vi "Mag Lab Init Device List.vi"(8 "error in (no error)":errorcluster) -> (0 "error out":errorcluster, 2 "find list":refnum<visa-resource-name>[](array[refnum]), 3 "Found Array":refnum<class "Mag Lab Hardware.lvclass">[](array[class]))   [LabVIEW 2015]
uses:
  Mag Lab Hardware.lvclass
  <vilib>/Instr/_visa.llb/VISA Find Search Mode.ctl
panel:
  out "Names":string[](array[string])
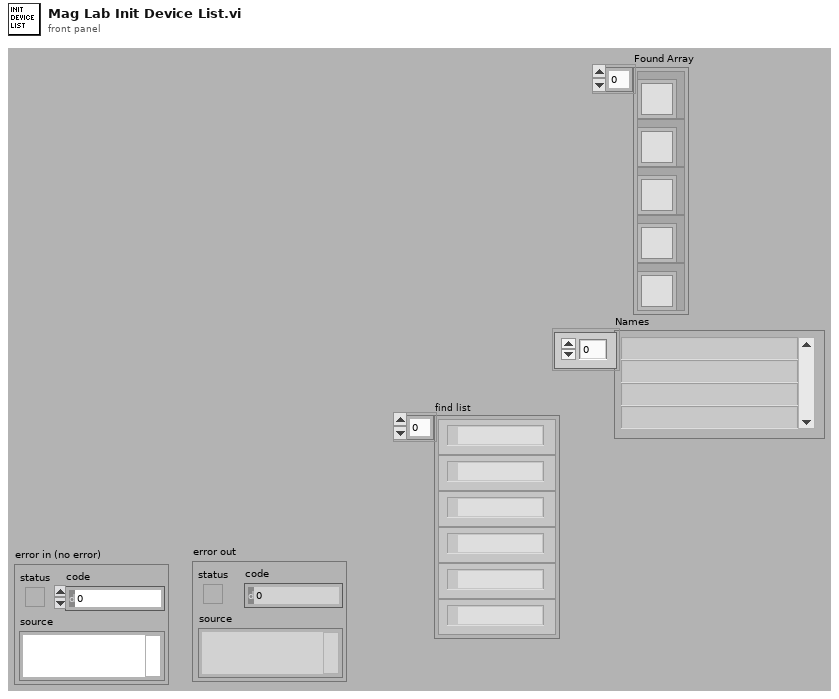
[diagram p1: front panel]
types:
  T1 = typedef "VISA Find Search Mode.ctl" = u32
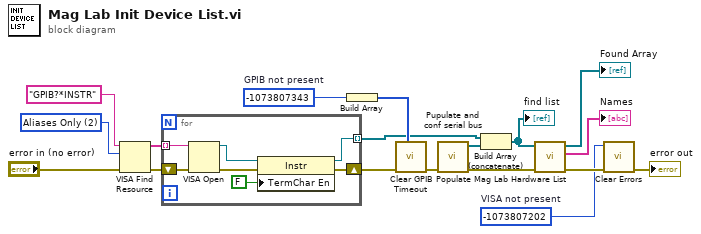
[diagram p0: block diagram]
diagram:
  w1 = -1073807202  # VISA not present
  w13 = -1073807343  # GPIB not present
  w17 = T1 2 items=["Canonical Names Only"=0, "Aliases Only"=2, "Include Matching Aliases"=3, "Include All Aliases"=4] ("Search Mode")
  n1 = VISA Find Resource(8:"error in (no error)", 10:w17, 11:"GPIB?*INSTR" ("expression (\"?*\")")) -> (0:w7:errorcluster, 3:w5:string[])  [unwired: 1 out]
  n2 = for {
    shift-right: [w21] -> w6
    shift-left: w7 -> [w23]
    tunnel: w5 -> [w25] mode=indexing
    tunnel: [w20] -> w4 mode=indexing
    n3 = VISA Open(error in (no error)=w23, VISA resource name=w25) -> (VISA resource name=w24:refnum<visa-resource-name>, error out=w22:errorcluster)  [unwired: 3 in]
    n4 = property class="Instr"(reference=w24, error in=w22, "TermChar En"=FALSE ("Message Based Settings:Termination Character Enable")) -> (reference out=w20:refnum<visa-resource-name>, error out=w21:errorcluster)
  }
  n5 = Build Array(w13) -> (w12:i32[])
  n6 = call "Clear GPIB Timeout.vi"("Errors to skip"=w12, "error in (no error)"=w6) -> ("error out"=w11:errorcluster)  [unwired: 9 out]
  n7 = call "Pupulate and conf serial bus.vi"("Error In"=w11) -> ("Error Out"=w10:errorcluster, "Devices"=w15:refnum<visa-resource-name>[])  [unwired: 9 in]
  n8 = Build Array (concatenate)(w4, w15) -> (w14:refnum<visa-resource-name>[])
  "find list" <- w14
  n9 = call "Populate Mag Lab Hardware List.vi"("error in (no error)"=w10, "VISA Resourse Names"=w14) -> ("error out"=w9:errorcluster, "Names"=→"Names":string[], "Instrument List"=→"Found Array":refnum<class "Mag Lab Hardware.lvclass">[])  [unwired: 7 in]
  n10 = call <vilib>:"Clear Errors.vi"("error in (no error)"=w9, "specific error code to clear (0: all)"=w1) -> ("error out"=→"error out":errorcluster)  [unwired: 4 in, 1 out]
